vi "Terminal-Alert-6220.vi"(11 "6220":T1) -> (3 "6220输出":T1)   [LabVIEW 2014]
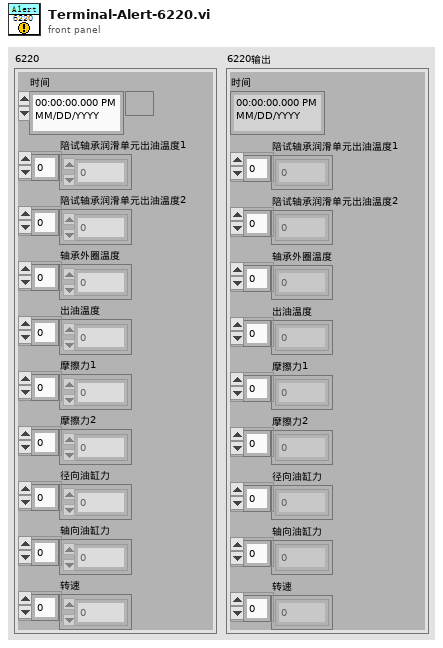
[diagram p1: front panel]
types:
  T1 = cluster{"时间":timestamp, "陪试轴承润滑单元出油温度1":sgl[], "陪试轴承润滑单元出油温度2":sgl[], "轴承外圈温度":sgl[], "出油温度":sgl[], "摩擦力1":sgl[], "摩擦力2":sgl[], "径向油缸力":sgl[], "轴向油缸力":sgl[], "转速":sgl[]}
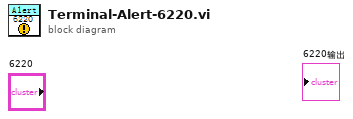
[diagram p0: block diagram]
diagram:
